vi "Read Record.vi"(8 "error in (no error)":errorcluster, 11 "Sim Configuration Database Actor in":refnum<class "Sim Configuration Database Actor.lvclass">) -> (0 "error out":errorcluster, 3 "Sim Configuration Database Actor out":refnum<class "Sim Configuration Database Actor.lvclass">)   [LabVIEW 2019, in "Sim Configuration Database Actor.lvlib" / "Sim Configuration Database Actor.lvclass"]
uses:
  Sim Configuration Database Actor.lvclass
  C:/Program Files (x86)/National Instruments/LabVIEW 2019/vi.lib/ActorFramework/Actor/Actor.lvclass
  <vilib>/ActorFramework/Actor/Actor.lvclass/Actor.ctl
  Sim Configuration Database Actor.lvclass/Sim Configuration Database Actor.ctl
  Car Wash Controller/Car Wash Controller Messages/Get DB Record Msg/Get DB Record Msg.lvclass/Get DB Record Msg.ctl
  <vilib>/ActorFramework/Message Enqueuer/Message Enqueuer.lvclass/Message Enqueuer.ctl
  Car Wash Controller/Car Wash Controller Messages/Set Timing Msg/Set Timing Msg.lvclass/Set Timing Msg.ctl
  <vilib>/ActorFramework/Message Enqueuer/Enqueue.vi
  Car Wash Controller/Car Wash Controller Messages/Get DB Record Msg/Get DB Record Msg.lvclass
  C:/Program Files (x86)/National Instruments/LabVIEW 2019/vi.lib/ActorFramework/Message/Message.lvclass
  Car Wash Controller/Car Wash Controller Messages/Set Timing Msg/Set Timing Msg.lvclass
  <vilib>/ActorFramework/Message Priority Queue/Priority Enqueue.vi
  <vilib>/ActorFramework/Actor/Actor.lvclass
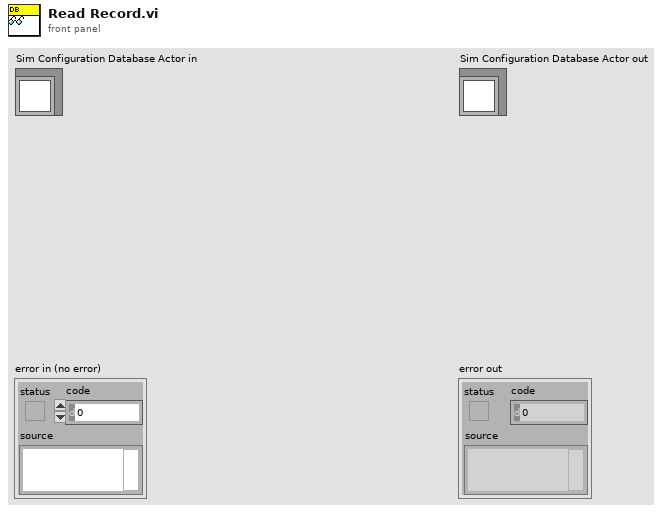
[diagram p1: front panel]
types:
  T1 = typedef "Sim Configuration Database Actor.lvlib/Sim Configuration Database Actor.lvclass/Record.ctl" = cluster{"Wash Step":string, "Step Duration":dbl, "Station":T2}
  T2 = typedef "Vehicle Position Sinmulation Actor.lvlib/Vehicle Position Simulation Actor.lvclass/Station -Enum.ctl" = enum16{"Entry", "Station1", "Station2", "Station3", "Exit"}
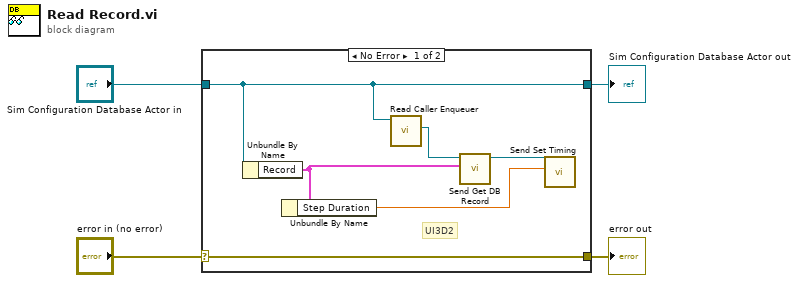
[diagram p0: block diagram]
diagram:
  n1 = case shown="No Error" "error in (no error)" {
    selector: "error in (no error)" -> [w10 w11]
    tunnel: [w10 w11] -> w3
    tunnel: [w9 w12] -> w1
    tunnel: "Sim Configuration Database Actor in" -> [w9 w12]
    frame No Error {
      # "UI3D2"
      n2 = Unbundle By Name(w9) -> ("Record"=w6:T1)
      n3 = Unbundle By Name(w6) -> ("Step Duration"=w5:dbl)
      n4 = call <vilib>:"Read Caller Enqueuer.vi"("Actor"=w9) -> ("Caller Enqueuer"=w8:refnum<class "Message Enqueuer.lvclass">)  [unwired: 10 in]
      n5 = call "Send Get DB Record.vi"("Record"=w6, "Message Enqueuer"=w8) -> ("Message Enqueuer out"=w7:refnum<class "Message Enqueuer.lvclass">)  [unwired: 8 in, 1 out]
      n6 = call "Send Set Timing.vi"("Timing Remaining"=w5, "Message Enqueuer"=w7) -> ()  [unwired: 8 in, 2 out]
    }
    frame Error {
    }
  }
  "error out" <- w3
  "Sim Configuration Database Actor out" <- w1
